vi "MED_CORR_FASE.vi"(0 "Seleción método":bool, 1 "Ejecucion":bool, 2 "Directorio scripts matlab":path=path "C:/Users/franjas/Documents/rutinas-calibracion-slm") -> ()   [LabVIEW 2013]
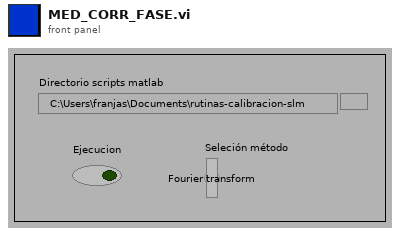
[diagram p1: front panel]
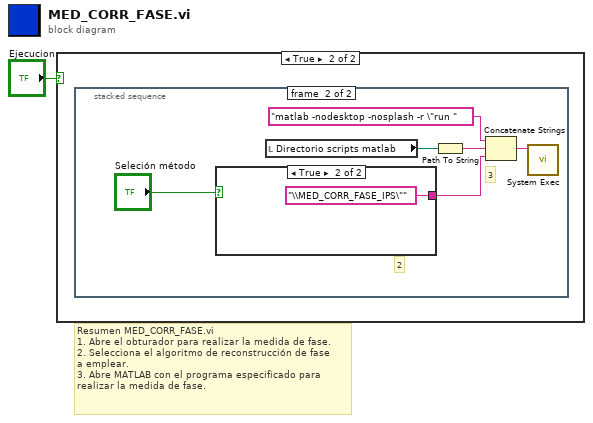
[diagram p0: block diagram]
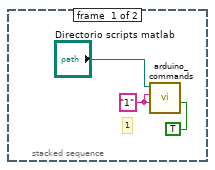
[diagram p3: hidden frame]
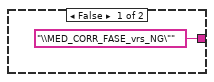
[diagram p4: hidden frame]
diagram:
  # "Resumen MED_CORR_FASE.vi\n1. Abre el obturador para realizar la medida de fase.\n2. Selecciona el algoritmo de reconstrucción de fase\na emplear.\n3. Abre MATLAB con el programa especificado para\nrealizar la medida de fase."
  n1 = case shown="True" "Ejecucion" {
    frame False {
    }
    frame True {
      n2 = stacked-sequence {
        frame #0 {
          w3 = "1" ("Número de motor")
          # "1"
          n3 = call "arduino_commands.vi"("Shutter on"=TRUE, "Argumento"=w3, "Número de motor"=w3, "Directorio scripts ArduinoStepper.py"="Directorio scripts matlab") -> ()  [unwired: 7 in, 1 out]
        }
        frame #1 {
          # "2"
          # "3"
          n4 = case shown="True" "Seleción método" {
            tunnel: ["\\MED_CORR_FASE_vrs_NG\"" ("command line") "\\MED_CORR_FASE_IPS\"" ("command line")] -> w7
            frame False {
            }
            frame True {
            }
          }
          n5 = local read "Directorio scripts matlab"() -> (w5:path)
          n6 = Path To String(path=w5) -> (string=w8:string)
          n7 = Concatenate Strings("matlab -nodesktop -nosplash -r \"run " ("command line"), w8, w7) -> (w9:string)
          n8 = call <vilib>:"System Exec.vi"("command line"=w9) -> ()  [unwired: 7 in, 4 out]
        }
      }
    }
  }
